vi "Test Base Clear Method is Called.vi"(8 "error in (no error)":errorcluster, 11 "Base Class Test in":refnum<class "Base Class Test.lvclass">) -> (0 "error out":errorcluster, 3 "Base Class Test out":refnum<class "Base Class Test.lvclass">)   [LabVIEW 2020, in "Base Class Test.lvclass"]
uses:
  Base Class Test.lvclass
  C:/Program Files (x86)/National Instruments/LabVIEW 2020/vi.lib/Asteme/LUnit/Test Case.lvclass
  Base Class Test.lvclass/Base Class Test.ctl
  <vilib>/Asteme/LUnit/Test Case.lvclass/Test Case.ctl
  <vilib>/Asteme/LUnit/LUnit Assertion Result.lvclass/LUnit Assertion Result.ctl
  <vilib>/Asteme/LUnit/Palette/Fail.vi
  <vilib>/Asteme/LUnit/Palette/Pass.vi
  <vilib>/Asteme/LUnit/Set Assertion Type.vi
  <vilib>/Asteme/LUnit/Add test result.vi
  <vilib>/Asteme/LUnit/LUnit Write Passed.vi
  <vilib>/Asteme/LUnit/LUnit Get Test Case.vi
  <vilib>/Asteme/LUnit/LUnit Write Message.vi
  <vilib>/Asteme/LUnit/LUnit Write Description.vi
  <vilib>/Asteme/LUnit/LUnit Write Assertion Type.vi
  <vilib>/Asteme/LUnit/Read Test Case Name.vi
  <vilib>/Asteme/LUnit/Assertion Result/LUnit Get Test Name.vi
  Framework/Base/Base.lvclass
  <vilib>/Asteme/LUnit/LUnit Assertion Result.lvclass
  <vilib>/Asteme/LUnit/Test Case.lvclass
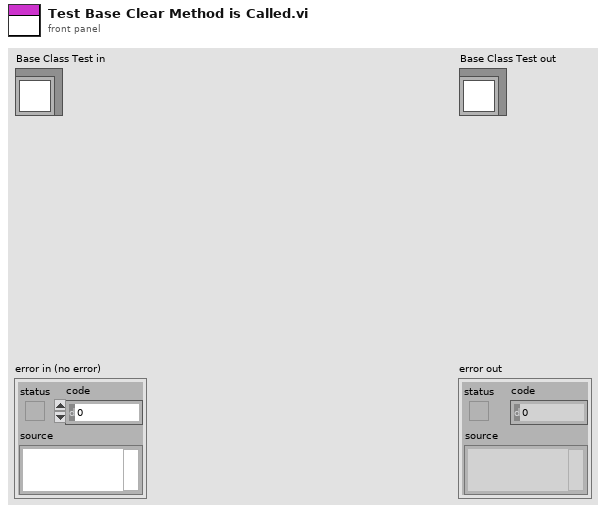
[diagram p1: front panel]
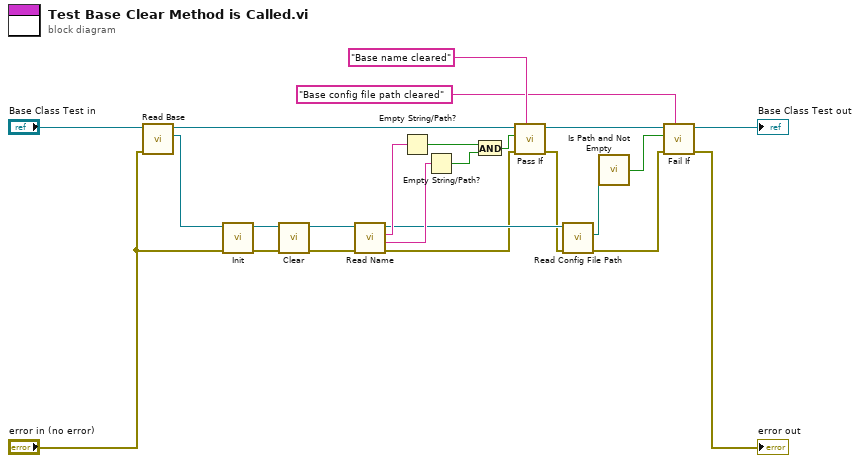
[diagram p0: block diagram]
diagram:
  n1 = call "Read Base.vi"("error in (no error)"="error in (no error)", "Base Class Test In"="Base Class Test in") -> ("Base.lvclass"=w18:refnum<class "Base.lvclass">, "Base Class Test Out"=w23:refnum<class "Base Class Test.lvclass">)  [unwired: 7 in, 1 out]
  n2 = call-dynamic "Init.vi"("error in (no error)"="error in (no error)", "Base In"=w18) -> ("error out"=w22:errorcluster, "Base Out"=w21:refnum<class "Base.lvclass">)  [unwired: 8 in]
  n3 = call-dynamic "Clear.vi"("error in (no error)"=w22, "Base In"=w21) -> ("error out"=w19:errorcluster, "Base Out"=w20:refnum<class "Base.lvclass">)  [unwired: 8 in]
  n4 = call-dynamic "Read Name.vi"("error in (no error)"=w19, "Base In"=w20) -> ("error out"=w8:errorcluster, "Name"=w14:string, "Qualified Name"=w15:string, "Base Out"=w10:refnum<class "Base.lvclass">)  [unwired: 6 in]
  n5 = Empty String/Path?(string/path=w15) -> (empty?=w13:bool)
  n6 = Empty String/Path?(string/path=w14) -> (empty?=w11:bool)
  n7 = And(x=w13, y=w11) -> (x .and. y?=w12:bool)
  n8 = call <vilib>:"Pass If.vi"("Description"="Base name cleared", "error in (no error)"=w8, "Pass?"=w12, "Test Case In"=w23) -> ("error out"=w9:errorcluster, "Test Case Out"=w7:refnum<class "Base Class Test.lvclass">)  [unwired: 6 in]
  n9 = call-dynamic "Read Config File Path.vi"("error in (no error)"=w9, "Process In"=w10) -> ("error out"=w3:errorcluster, "Config File Path"=w5:path)  [unwired: 7 in, 1 out]
  n10 = call <vilib>:"Is Path and Not Empty.vi"("path"=w5) -> ("Is Path and Not Empty?"=w4:bool)  [unwired: 4 in]
  n11 = call <vilib>:"Fail If.vi"("Description"="Base config file path cleared", "error in (no error)"=w3, "Fail?"=w4, "Test Case In"=w7) -> ("error out"=→"error out":errorcluster, "Test Case Out"=→"Base Class Test out":refnum<class "Base Class Test.lvclass">)  [unwired: 6 in]
